vi "RockPaperScissors - 2.vi"() -> ()   [LabVIEW 2021]
panel:
  out "sum":i32
  out "array":string[][](array[string])
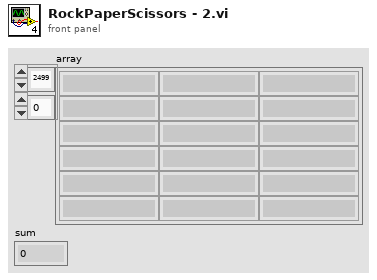
[diagram p1: front panel]
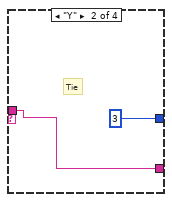
[diagram p3: hidden frame]
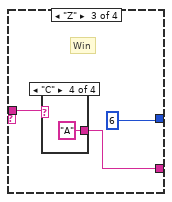
[diagram p4: hidden frame]
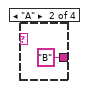
[diagram p6: hidden frame]
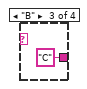
[diagram p7: hidden frame]
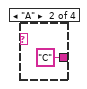
[diagram p9: hidden frame]
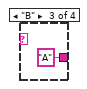
[diagram p10: hidden frame]
diagram:
  w6 = map{string, i32} {}  # Size: 0
  w12 = "%s" ("format string")
  n1 = Build Array(w12) -> (w11:string[])
  n2 = Build Array(w11) -> (w10:string[][])
  n3 = for {
    shift-right: [w13] -> w3
    shift-left: w6 -> [w16]
    tunnel: string[] ["A", "B", "C"] -> [w15] mode=indexing
    tunnel: i32[] [1, 2, 3] -> [w14] mode=indexing
    n4 = Insert Into Map(map in=w16, key=w15, value=w14) -> (map out=w13:map{string, i32})  [unwired: 2 out]
  }
  n5 = Spreadsheet String To Array(delimiter (Tab)=" ", format string=w12, spreadsheet string="C X\nA Y\nC Z\nB Y\nC Z\nA Z\nB Y\nC Z\nC Z\nB X\nA X\nA Z\nC Z\nC X\nA Z\nA Z\nC Z\nA X\nA Z\nA Z\nA Z\nA Z\nA Z\nC Z\nA Z\nC X\nC Z\nA Z\nA Z\nB Y\nC Z\nB X\nB X\nA Z\nC Z\nA X\nA X\nB Y\nB Z\nB Y\nA Z\nC Z\nC X\nC Z\nC Z\nC Z\nC Z\nA Z\nA Z\nA Y\nA Y\nC Z\nA X\nC Y\nA Z\nB Y\nC Z\nC Z\nB Y\nC Z\nC Z\nC Z\nA Z\nA Z\nB Y\nC Z\nA Z\nC Z\nC Z\nA Z\nB X\nC Z\nA X\nA X\nA Y\nC X\nA Y\nB X\nA Z\nA Z\nC Z\nA Z\nA Y\nC X\nA X\nB Y\nA Z\nA Y\nC Z\nC Y\nA X\nB Z\nB Y\nA Y\nC Z\nC Z\nC Z\nB Y\nA Z\nC Z\nA Y\nC Z\nA X\nC Z\nC Z\nA Z\nA X\nC X\nC X\nA X\nA X\nA Y\nA Z\nC Z\nA X\nA Z\nB Y\nA Y\nA Z\nC Z\nB Y\nA Z\nC Z\nA Z\nA X\nA Z\nB Y\nC Z\nC Z\nC Z\nC X\nA X\nC Z\nA X\nB Y\nC X\nC Z\nB Y\nB Y\nB X\nC Z\nB Y\nC Z\nC Z\nC Z\nA Z\nC Z\nC Z\nB Y\nC Z\nB Z\nC Z\nC Z\nA X\nC Z\nC Z\nA Z\nC Z\nC X\nC Z\nA Z\nA Z\nA X\nB X\nC Y\nA X\nA Y\nC Y\nC Z\nA Z\nA X\nC X\nC Z\nA X\nB Y\nC Z\nA X\nA X\nC Z\nB Y\nC Z\nA Y\nA Z\nB Y\nA Y\nA X\nC X\nA Z\nC Z\nB Y\nC Z\nC Z\nC Z\nC Z\nA Z\nC Y\nC Z\nA Y\nA X\nA Z\nA Z\nA Z\nC Z\nC Z\nA Z\nC Z\nA Z\nC Z\nA Z\nC Z\nA X\nB Y\nC Z\nC Z\nC X\nB X\nA Z\nC Z\nA Y\nC Z\nB Y\nA Z\nC Y\nC Z\nC Y\nC Z\nB Y\nA Y\nA Z\nC Z\nC X\nC Z\nA Z\nA Z\nA Z\nA Z\nA Z\nC Z\nC X\nA X\nC Z\nA X\nA Z\nA Z\nA Z\nA Z\nA Z\nB Y\nC Z\nC Z\nA Z\nC Z\nC Z\nC Z\nA Z\nC Z\nC Z\nB Y\nC Z\nA Z\nA Y\nC Y\nB Y\nA Z\nA X\nA Y\nC X\nB Y\nC Z\nC X\nC Z\nA Z\nB Y\nC Z\nC X\nC Z\nA Y\nB Z\nC Z\nC Z\nC Z\nA X\nB Y\nC Z\nC X\nB Y\nB Y\nC X\nA Z\nB Y\nC Z\nA X\nB Y\nC Z\nC Z\nA Z\nB Y\nB Y\nB Y\nA X\nC Z\nB Y\nB Y\nB Y\nA X\nA Z\nC Z\nC Z\nB Y\nA Z\nB Y\nB X\nA Z\nC X\nA Z\nC Z\nA Z\nC Y\nA X\nB Y\nC Z\nB Y\nC Y\nC X\nA Y\nC Z\nA Y\nC X\nA Z\nA Z\nA Z\nA Z\nC Z\nA Y\nB Y\nC Z\nC Z\nB Y\nC Z\nC Z\nC Z\nC Z\nC Z\nC Z\nA X\nC Z\nC Z\nC Z\nA X\nA Z\nA X\nA Z\nA X\nA X\nC Z\nA Z\nB Y\nC Z\nA Z\nC Y\nA Z\nB Y\nB Y\nC Z\nB Y\nB Y\nA Y\nB Y\nA X\nC Z\nA Y\nC Z\nA Z\nA Z\nA X\nA Z\nA X\nC Z\nB Y\nA Z\nA X\nC Z\nC Z\nC Z\nA Z\nA Z\nC X\nA Z\nA Y\nA X\nC Z\nA Y\nC Z\nB X\nC X\nA X\nA X\nC Z\nA Y\nC X\nA Z\nB X\nA Z\nA Z\nA Z\nA X\nA Y\nA Z\nC Z\nA X\nC Z\nA X\nA Z\nA Z\nB Y\nA Z\nC X\nC X\nC Z\nA Z\nC X\nA Z\nA Y\nC Z\nC Z\nB Y\nC Z\nC Z\nA Z\nA Y\nB X\nC X\nC Z\nA Z\nC Z\nA X\nA Z\nA Z\nB Y\nA Y\nA Z\nA Z\nA Z\nC Y\nB Y\nA Y\nC Z\nC Z\nC X\nB Y\nC Z\nC Z\nA Y\nA X\nC Z\nC Z\nC X\nA Z\nB X\nC Z\nB Y\nA Y\nC Z\nC Z\nB X\nA X\nA X\nC Z\nA X\nA X\nC Z\nA Z\nC Z\nA Z\nA Z\nC Z\nA Y\nC Z\nC Z\nC Z\nA Z\nC Z\nC Z\nA Y\nC Z\nC Z\nC Z\nC Z\nC Z\nA Z\nC Z\nB Y\nA Z\nC Z\nC X\nA X\nC Z\nB Y\nA Z\nA X\nB Y\nC Z\nC Z\nC Z\nA X\nC Z\nA Z\nA Y\nA Y\nA Z\nA Z\nA Y\nB Y\nA Z\nC Z\nB Y\nC Z\nA Z\nC Z\nB Y\nB Z\nA X\nC Z\nA Y\nA Y\nA Z\nA X\nC Z\nC Z\nC Z\nC Z\nC Z\nA Z\nC Z\nA Z\nA Y\nA Z\nC X\nA Z\nC Y\nB Z\nC X\nA Z\nA X\nA X\nB Y\nC X\nC Z\nB Y\nA Z\nC Z\nC Z\nA Z\nC Z\nA Z\nC X\nC Y\nC Z\nA X\nC Y\nC Z\nA Z\nA Z\nC Z\nC Z\nA Y\nC Z\nC Z\nB Z\nC X\nA X\nA Z\nC Z\nA Y\nC Z\nC Z\nA X\nA Z\nA X\nA Y\nA Y\nA Y\nC Z\nB Y\nC Z\nA X\nC Y\nC Z\nB Y\nA X\nC Z\nA Z\nA Z\nB Y\nC Y\nA Y\nC Y\nA Z\nC Z\nA Z\nC Z\nC Z\nA Z\nA Z\nC Z\nA Z\nC Z\nA Y\nC Z\nC X\nC Z\nC Z\nC Z\nC Z\nA X\nB Z\nB X\nB Y\nB Y\nC Z\nA X\nA X\nB Y\nA Z\nA X\nC Z\nA X\nC X\nA Y\nA X\nC Z\nC Z\nC Z\nC Z\nC Z\nA X\nC Z\nB Y\nC X\nA X\nA Z\nA Z\nC Z\nC Z\nA Z\nA Z\nC Z\nA X\nA Z\nB Y\nC X\nA X\nA Y\nA Z\nC Z\nA Z\nA Z\nB Y\nA X\nB Y\nC X\nA Y\nB Y\nA Z\nC Z\nB Y\nA Z\nC Z\nC Z\nA Z\nC Z\nA Z\nC Z\nB Y\nA Z\nA Y\nC Z\nB Y\nA Z\nC Z\nC Z\nA Z\nA X\nA Z\nA Z\nC Y\nA Y\nC Z\nC Y\nC Z\nC Z\nB Y\nC Z\nC Y\nA Z\nC Z\nB Z\nC Y\nB Y\nC Y\nC Z\nA Y\nC Z\nA Z\nC Z\nA Y\nC Z\nC Z\nB Y\nB Y\nA Z\nC Z\nB Z\nC X\nB Y\nB Y\nC X\nB Y\nA X\nA X\nA Y\nA Z\nA X\nA X\nC Z\nC Z\nC Z\nC X\nC Z\nB Y\nB Z\nC Z\nA Z\nA Y\nA X\nB Y\nB X\nA X\nA Z\nC Z\nC Z\nA Z\nC Z\nA X\nB X\nB Z\nC Z\nB Y\nA Z\nA Z\nC X\nA X\nA Y\nC Z\nB Y\nC Z\nA Z\nA Z\nA Y\nC Z\nA Z\nA Z\nA Z\nC Z\nC Z\nC Z\nA X\nA X\nB X\nC Z\nA Y\nA Y\nA Y\nC Z\nA Z\nA X\nC Z\nA Z\nA Z\nA X\nC Z\nC Z\nC X\nA Z\nC Z\nC Z\nC Z\nA Z\nC Z\nA Z\nC X\nA Z\nC Z\nC Z\nA Y\nA Y\nC Z\nC Z\nC X\nA Z\nA Y\nC Z\nB Y\nC Z\nA Z\nC Z\nC X\nA Z\nA X\nB Y\nB Y\nC Z\nA Z\nA Z\nA Z\nB Z\nB Y\nC Z\nA Z\nC Z\nC Z\nA Z\nA Z\nA Z\nA X\nB Y\nC Z\nA X\nA Y\nA Z\nC Z\nA Z\nC Z\nC Z\nC X\nA Y\nC Z\nC Z\nC Z\nC Z\nB Y\nC Z\nC Z\nB Z\nC Z\nA X\nC Z\nC Z\nC Z\nA Z\nC Z\nC X\nA Y\nC Z\nA Z\nA Y\nA X\nB X\nB Y\nA Z\nA Z\nA X\nA Z\nC Z\nA Z\nA Z\nA Z\nA Z\nC Z\nA X\nA Z\nA Z\nA Y\nC Z\nB Y\nA X\nA X\nA X\nB Y\nC Z\nC Z\nC Z\nC Z\nB Y\nA X\nC Z\nB Y\nA Z\nC Z\nA Z\nB X\nB Y\nA X\nC Z\nC Z\nC X\nA Z\nA X\nC Z\nB Z\nA X\nA Z\nC Y\nA X\nC Z\nA X\nC Z\nC Z\nA Y\nA Z\nB Y\nA Z\nC X\nA Y\nC Z\nC Z\nA Y\nA Z\nC Z\nA Y\nA X\nA X\nA Y\nC Z\nC Z\nC Z\nA Z\nA Z\nC X\nA Z\nC Z\nA X\nC Z\nB Y\nC Y\nC Z\nA Z\nC Z\nA Z\nA Z\nC Z\nC Z\nA Z\nC Z\nC X\nA Z\nB Y\nA Y\nC Z\nC Z\nC Z\nC Z\nB Y\nA Z\nA Z\nA Z\nC Z\nA X\nC Z\nA Z\nC Y\nC X\nC Z\nC Z\nC Z\nA X\nB Y\nA X\nC Y\nC Y\nA Z\nA Z\nB Y\nA Y\nA Z\nA X\nC Z\nA Z\nC Z\nC Z\nA Z\nA X\nA Z\nA Z\nA Z\nC Z\nC Z\nA Z\nC Z\nA Z\nB Y\nA Z\nC Z\nA Y\nB Y\nB Y\nC Z\nA X\nA X\nC X\nB X\nB Y\nC Z\nB Y\nC Z\nC Z\nB Y\nC Z\nA Z\nA Y\nC Z\nC Z\nC Z\nB Y\nC Z\nC Y\nC Z\nA Z\nA Z\nB Y\nA X\nA X\nC Z\nB Y\nC X\nC Z\nA Z\nC Z\nC Z\nA X\nA Z\nA X\nC Z\nB Y\nC Z\nC Z\nC Z\nC Z\nA Z\nA Y\nC Z\nC X\nA Y\nA X\nA X\nA X\nC X\nA Z\nB Y\nB X\nC Z\nA Z\nC Z\nC Y\nA Z\nB Y\nA X\nA Z\nA Y\nC Z\nA Z\nA Z\nA X\nC Y\nA Z\nC Z\nA X\nB Y\nC Z\nA Y\nC Z\nC Z\nB Y\nA Y\nC Z\nA X\nA X\nA Y\nC X\nA X\nC X\nC X\nC Z\nA X\nC Z\nC Y\nC Z\nC X\nB Y\nC Z\nC Y\nA X\nC Z\nA X\nB Z\nA Y\nA Z\nC Z\nC Z\nC Z\nC Z\nA X\nC Z\nC Z\nC Z\nA Z\nB Y\nC Z\nC X\nB Y\nA Z\nC Z\nB Z\nC Z\nA Z\nC Z\nA Z\nB Y\nA Z\nC Z\nC Z\nC X\nA X\nA Z\nB Y\nC Z\nA X\nA Z\nA X\nB Y\nC Z\nA X\nC Z\nC Z\nC X\nC Z\nC Z\nC Z\nA X\nC Z\nB Z\nA Z\nB Y\nC Z\nB Z\nC X\nC X\nC Z\nC Z\nC Z\nB X\nC Z\nC Z\nC Z\nA Z\nB X\nA Y\nA Z\nC Z\nA Y\nA Z\nA X\nA Z\nA Y\nA X\nA Z\nA Z\nC Z\nC Z\nC Z\nA Y\nA X\nA Y\nB Y\nC Z\nB Y\nC Z\nC Z\nA X\nC X\nA Z\nC Z\nB Y\nA Z\nC Z\nB X\nA Y\nC Z\nC Z\nA Y\nC Z\nC Z\nA X\nC Y\nC Z\nA Z\nA Z\nA X\nA Y\nA Z\nC Z\nC Z\nA Z\nA X\nC Z\nA Y\nB X\nB X\nA Z\nA Z\nC Z\nA X\nA X\nC Z\nC X\nC Z\nC Z\nC Z\nC Z\nC X\nC X\nC Z\nA Y\nC Z\nC Z\nC Z\nA X\nB Y\nA Z\nC Z\nA Y\nA Y\nA Z\nC Z\nC Z\nA Z\nA Y\nA Z\nC Z\nC Z\nB X\nA X\nC Z\nC Z\nA Z\nC Z\nA Z\nC Z\nA Z\nA X\nA X\nA Z\nA X\nC Z\nC X\nA Z\nC X\nB Y\nA X\nA Z\nA Z\nC Z\nA Y\nA X\nC X\nA Z\nC X\nC Z\nA X\nC Z\nC Z\nB Y\nB Y\nC Z\nC X\nB Y\nA Z\nC Z\nC Z\nC Y\nC Z\nC Y\nC Z\nA X\nA Y\nB X\nC Z\nB Y\nA Y\nA X\nC X\nA Z\nA Y\nC Z\nB Y\nA Y\nC X\nA Z\nA Y\nA X\nC Z\nC Z\nC Z\nC Z\nA X\nA Y\nB Y\nC Z\nC Y\nA X\nA X\nA Z\nA Z\nA Z\nA Z\nA Z\nC Z\nA Z\nC Y\nA Y\nA Y\nB Y\nA Z\nA Z\nA Y\nC Z\nC Z\nA Z\nB Y\nB Y\nC Z\nB Y\nA X\nB Y\nA Y\nB Y\nC X\nB Y\nA X\nB Z\nC Z\nC Z\nC Z\nC Z\nA Y\nC Z\nA Z\nA Y\nB Y\nA X\nC Z\nB X\nC Z\nC Z\nC Z\nA Z\nA Z\nA Z\nA X\nC Y\nA Z\nB Y\nC Z\nC Z\nC Z\nA X\nB Y\nB Z\nC Z\nC Z\nC X\nA Z\nA X\nA X\nC Z\nA Z\nA X\nC Z\nA X\nA Z\nA Y\nC Z\nA Y\nC X\nA Z\nA X\nA Z\nC Z\nB Z\nA Y\nA X\nC X\nC Y\nB Y\nA X\nC Z\nC Z\nC Z\nC X\nC Z\nC X\nC Z\nC Z\nA Z\nA Z\nB Y\nA Y\nC X\nA X\nC Z\nA X\nC Z\nC Z\nB Y\nA Z\nA Y\nB Y\nA X\nC Z\nA Y\nA Z\nC Z\nB Y\nA X\nC Z\nB Y\nC Z\nA Z\nB Y\nC Y\nC X\nB Z\nA Z\nC Z\nA Z\nA Y\nC Z\nA Z\nC Z\nC Z\nC Z\nA Y\nC Z\nC Z\nA Z\nB Z\nC Z\nC Z\nC X\nA Z\nC X\nB X\nC X\nA Y\nC Z\nA Z\nA Y\nC X\nA X\nB Y\nC Y\nA Z\nA Z\nC Y\nC X\nA X\nA Z\nC Z\nA X\nA Z\nC X\nA X\nB X\nC Z\nC Z\nA X\nC X\nA Z\nA Z\nA Y\nC Z\nA X\nB Y\nC Z\nA Z\nC X\nA X\nC Z\nB Y\nA X\nB Y\nA Y\nC Y\nA Y\nC Y\nA X\nA Z\nC Z\nB Y\nC Z\nC Z\nB Y\nA X\nA Y\nB Y\nA X\nB X\nA Z\nC Z\nC X\nA Z\nA X\nC Z\nA Y\nC Z\nA Z\nA Z\nA Z\nA Y\nA Z\nB Y\nC Z\nC X\nC X\nC Z\nA Z\nA Z\nA X\nB Y\nC Z\nA Z\nC X\nB X\nC Z\nC Z\nA Z\nC Z\nC Z\nA Z\nB Y\nA X\nB X\nB Y\nA Z\nA Z\nA Z\nA Z\nA Y\nC Z\nC Z\nC Y\nB Y\nB Y\nB Y\nC Z\nC Z\nA X\nA Y\nC Z\nB Y\nB Z\nA X\nC Y\nC Z\nA X\nC Z\nC X\nA X\nC Z\nC Z\nA Y\nA X\nA Z\nA Z\nA Y\nC Z\nA Z\nC X\nB Z\nC Z\nB Y\nA Y\nC Z\nC Z\nA X\nC Z\nC X\nC X\nA Z\nA Y\nA Y\nB Y\nC X\nC Z\nA Z\nC X\nB Y\nA Z\nC Z\nA Y\nC Z\nA Z\nC Z\nA X\nC X\nA X\nA X\nA Y\nB Y\nC Z\nC Z\nA X\nC Z\nA Y\nA Z\nA Y\nB Y\nC Z\nA Z\nA Z\nA Z\nA Y\nC Y\nB X\nA X\nC Z\nA Y\nC Z\nA Y\nB Z\nA X\nC Z\nA Z\nC Z\nA Z\nA X\nC X\nA X\nA X\nA Z\nA Z\nC X\nB Y\nC Z\nC Y\nA Z\nA Z\nA Z\nA Z\nA Z\nA X\nB Z\nB Y\nA Y\nC Z\nA Z\nB Y\nA Z\nC Y\nA Y\nA X\nC Z\nA Z\nC Z\nC Z\nC Y\nA Z\nC Z\nA X\nA Z\nA Z\nB Y\nC Z\nC Z\nC Z\nC Z\nC Z\nC Z\nC Z\nB Y\nC Z\nC Z\nA Z\nC Z\nB Y\nC X\nC X\nC Z\nC Z\nC Z\nA Z\nB Y\nA X\nC Z\nB Y\nB Y\nC Z\nA X\nC Z\nC X\nC Z\nB Y\nB Y\nC Z\nA Z\nC Z\nC X\nB Y\nC Z\nA Z\nC Z\nC Z\nC Z\nC Z\nA Y\nC Y\nA Y\nC Z\nC Z\nA X\nA Z\nC Y\nC Z\nA X\nB Z\nC X\nC Z\nA Z\nC Z\nC X\nC Z\nC Y\nA X\nA Z\nA Y\nA X\nB X\nA Z\nA Y\nA Z\nB Y\nA Z\nB Y\nB Y\nC Z\nA Z\nC Z\nC Z\nA X\nA X\nC Z\nC Z\nC Z\nC Z\nC X\nA Y\nC Z\nC Z\nA Z\nA Y\nC Z\nA Z\nB Y\nC Z\nC Z\nC Z\nC Z\nA Z\nB Y\nB Z\nB Z\nA Z\nA Y\nA X\nC Z\nB X\nC Z\nB Y\nA X\nC Y\nA Y\nC Z\nC Z\nC X\nC Z\nC X\nC X\nA Z\nA X\nA Z\nC Z\nB X\nA Z\nC Z\nC Z\nA Z\nA Y\nC X\nA X\nC Z\nA X\nA Y\nA X\nA X\nA Z\nA Z\nC Z\nA Z\nA Z\nA Z\nB Y\nA Z\nC Z\nA Y\nC Z\nC Z\nA Z\nA Y\nA Y\nC X\nA X\nB Z\nA Z\nC Z\nA Z\nA Y\nA X\nB Y\nB Y\nA Y\nA Z\nA Z\nB X\nC X\nA Z\nC Z\nC X\nC Z\nC Z\nA X\nC Z\nC Z\nB Y\nA Z\nA Z\nA Y\nA Z\nA Y\nC Z\nC Z\nC Z\nC Z\nB Y\nB Y\nA Z\nC Z\nA Z\nA X\nC Z\nC Z\nA Y\nC Z\nB Y\nA X\nA X\nA Z\nC Z\nC Z\nC Y\nC Z\nA X\nC Z\nA Z\nC Z\nB Y\nA Z\nC Z\nB Y\nB Y\nC Z\nA Y\nC Z\nC Y\nA Z\nA X\nA X\nC Z\nA Y\nC Z\nA Z\nC Z\nA X\nA X\nA Z\nA Z\nC Z\nB Y\nC X\nA Y\nC Z\nC Z\nA X\nC Y\nA Y\nC Z\nC Y\nA Z\nB Z\nC Z\nA Z\nB Y\nB Y\nA Z\nC Z\nA X\nA Z\nC Z\nA Z\nC Z\nC Z\nB Y\nB Y\nA X\nB Y\nA Z\nC Z\nA Z\nA Z\nC Z\nA Y\nC Y\nC Z\nA X\nC Z\nA Z\nC Z\nC Z\nC Y\nC Z\nA Z\nC Z\nC Z\nB Y\nA Z\nC Z\nB X\nB Y\nA Y\nC Z\nA Z\nB Y\nA Z\nC Z\nC X\nC Z\nA Y\nA Y\nA Y\nB Y\nC Z\nA Z\nA Z\nC Z\nA Z\nC X\nA Z\nA Z\nA X\nA Z\nA Y\nC Z\nA Z\nC Z\nA Z\nA X\nC Z\nC X\nC Z\nC Z\nC Z\nC Z\nC Z\nB Y\nC Z\nA Y\nC Z\nB Y\nC X\nC Z\nC Z\nC Z\nB X\nA X\nC Z\nC Z\nC X\nC Z\nA Y\nC Z\nA Z\nA Z\nC Z\nC Z\nC Z\nA Z\nC Z\nA X\nA Z\nC Z\nA Z\nC Z\nA X\nC Z\nC Z\nC X\nA Z\nC Z\nC Z\nC Z\nC Z\nA X\nA Z\nA X\nC Z\nB Y\nC X\nB Y\nA Z\nC Z\nC Z\nA X\nA Z\nA Y\nA X\nA Z\nB Z\nB Y\nC Z\nC Z\nA Y\nC Z\nB Y\nC Z\nB X\nA Z\nC Z\nA Y\nA Z\nA Z\nB Y\nC X\nA Y\nC Z\nC Z\nC Z\nB Z\nB Y\nB X\nA X\nA X\nC Z\nC Z\nC X\nA Y\nC Z\nC Z\nC Y\nC Z\nA Z\nA X\nC Z\nB Y\nC Y\nA Z\nC Z\nA X\nC Z\nC Z\nA X\nA Y\nC Z\nA Y\nC Z\nA X\nC Z\nC Z\nC Z\nC Y\nB Y\nA Z\nC Z\nC X\nB Y\nA Y\nB Y\nC Z\nC Z\nA X\nC Z\nC Y\nA Z\nA X\nA Y\nC Z\nB X\nB Y\nC Z\nA Z\nB Y\nA Y\nC Z\nA X\nB Y\nA X\nC Z\nA Z\nC Z\nB Y\nA Z\nC X\nB Y\nA Y\nA Z\nA Z\nA X\nB Y\nB Y\nC Z\nA X\nC X\nA Z\nB Y\nA X\nB Y\nC Z\nA Z\nA Z\nC Z\nC Z\nA Z\nA X\nC Z\nB Y\nC Z\nC Z\nA Z\nC Z\nA Z\nB Z\nA Z\nC Z\nA Z\nA X\nA X\nA X\nA Y\nC Z\nC Y\nC Z\nC Y\nA X\nA X\nA Y\nC Z\nA Y\nC Z\nC Z\nC X\nB Y\nC Z\nC Z\nC Y\nB Y\nA X\nB X\nA Z\nC Z\nB Y\nA Z\nB Y\nA Y\nA Z\nB Z\nA Y\nA Y\nA X\nA Z\nA Y\nB Y\nC Z\nA X\nC Z\nB Y\nA Z\nC Z\nA Z\nA X\nB Y\nC Z\nA Z\nA Y\nC X\nB Y\nC Z\nC X\nA X\nC Z\nA Y\nC Z\nA X\nB Y\nC Y\nC Z\nA Y\nC Z\nA Z\nA Z\nA Z\nC Z\nC X\nB Y\nB Z\nC Z\nC Z\nC Z\nA Z\nC Z\nC Z\nA Z\nA Z\nB Y\nC Z\nA X\nA Y\nA X\nA Y\nC Z\nC Z\nB Y\nA X\nA Z\nA Z\nA Z\nC Z\nB Z\nC Y\nC Z\nB Y\nC Y\nC Z\nA Z\nC Z\nC X\nA Z\nA Z\nB Y\nA Z\nC Z\nA Y\nA X\nA Z\nA Y\nC Z\nC Z\nB Y\nB Y\nC Z\nC Z\nC Z\nC X\nA Z\nA Z\nC Z\nB Y\nC X\nB X\nC Z\nA Z\nC Y\nC Z\nC Z\nA X\nC Z\nC Z\nC Z\nA Z\nA Y\nC Z\nB Y\nC Z\nA X\nB X\nC X\nC Z\nA Z\nC Z\nA Z\nA Z\nC Z\nA Y\nA Z\nC Z\nA Z\nA Z\nA X\nC X\nC X\nA X\nC Z\nB Y\nB Y\nA Z\nA Z\nA X\nA Y\nB Y\nC Y\nA Z\nA Z\nC Z\nA X\nC Z\nA Y\nB Y\nC X\nA Y\nC Z\nC Z\nC Z\nA Z\nA Z\nC Y\nA X\nA X\nA X\nC X\nC X\nA X\nC Z\nA X\nB Y\nA Z\nA Z\nC Z\nA X\nA X\nA X\nC Z\nC Z\nC Z\nA Z\nC Z\nA Z\nA Z\nA X\nA Y\nA Y\nC Z\nB Y\nA Y\nA Z\nB Y\nB Y\nC Z\nB Y\nA Y\nC X\nA Z\nA Y\nC Z\nC Z\nA X\nA Z\nB Y\nC Z\nA Y\nA Z\nA Z\nA Z\nC Z\nA Z\nB Y\nC Z\nA Z\nA Z\nA Z\nA Y\nA X\nB Y\nA Z\nA Z\nB X\nA Y\nC Z\nC Z\nA Z\nA Z\nB Y\nA Y\nC Z\nA Z\nC Z\nC X\nC Z\nC X\nC Z\nB Y\nA Y\nC Z\nB Y\nA X\nB Y\nB Y\nA Z\nC Z\nA X\nA X\nC Z\nA X\nA Z\nC Z\nC Z\nB Y\nA Z\nC Z\nC Z\nC Z\nC X\nA Z\nA Z\nC Z\nA Z\nC Z\nC Z\nC X\nB Y\nA X\nA Z\nA X\nC Z\nA Y\nC Z\nC Z\nA X\nC Z\nB X\nA Z\nA Z\nC Z\nC Z\nA Y\nA X\nA Z\nA Z\nC Z\nC Z\nC Z\nC Z\nC Z\nB Y\nA Y\nA Z\nC Z\nC Z\nC Z\nC Z\nC Z\nC X\nA Y\nC X\nC Z\nC Z\nA X\nA Z\nA Z\nC Z\nB Z\nA Z\nB Y\nA Z\nC Z\nC Y\nA Z\nC Z\nC Z\nA X\nC Z\nC Z\nB Y\nA Y\nB Y\nC Z\nA Z\nB X\nC Z\nA Y\nB Y\nC Y\nA Z\nA Y", array type (2D Dbl)=w10) -> (array=w7:string[][])
  "array" <- w7
  n6 = for {
    tunnel: w7 -> [w25] mode=indexing
    tunnel: w3 -> [w24]
    tunnel: [w20] -> w2 mode=indexing
    n7 = Index Array(array=w25) -> (element #1=w18:string, element #2=w19:string)  [unwired: 2 in]
    n8 = case shown="\"X\"" w19 {
      tunnel: [_ 3 ("default value") 6 ("default value") _] -> w22
      tunnel: w18 -> [_ w26 w29 w35]
      tunnel: [_ w26 w28 w34] -> w17
      frame Default {
      }
      frame "Y" {
        # "Tie"
      }
      frame "Z" {
        # "Win"
        n9 = case shown="\"C\"" w29 {
          tunnel: [_ "B" ("format string") "C" ("format string") "A" ("format string")] -> w28
          frame Default {
          }
          frame "A" {
          }
          frame "B" {
          }
          frame "C" {
          }
        }
      }
      frame "X" {
        # "Lose"
        n10 = case shown="\"C\"" w35 {
          tunnel: [_ "C" ("format string") "A" ("format string") "B" ("format string")] -> w34
          frame Default {
          }
          frame "A" {
          }
          frame "B" {
          }
          frame "C" {
          }
        }
      }
    }
    n11 = Look In Map(map=w24, key=w17, default value=0) -> (value=w21:i32)  [unwired: 1 out]
    n12 = Add(x=w22, y=w21) -> (x+y=w20:i32)
  }
  n13 = Add Array Elements(numeric array=w2) -> (sum=→"sum":i32)
